vi "En Setting for Trig and LSL.vi"(9 "LSL En enum":enum16{"LSL Disabled", "LSL Enabled"}(ring), 10 "Soft Trig enum":T1(ring), 11 "Data Cluster in":T2) -> (3 "Data Cluster out":T2)   [LabVIEW 2019, in "CML UI.lvlib"]
uses:
  CML UI.lvlib
  Module Data--cluster.ctl
  Acquisition State.ctl
  Measurement UI Displays.ctl
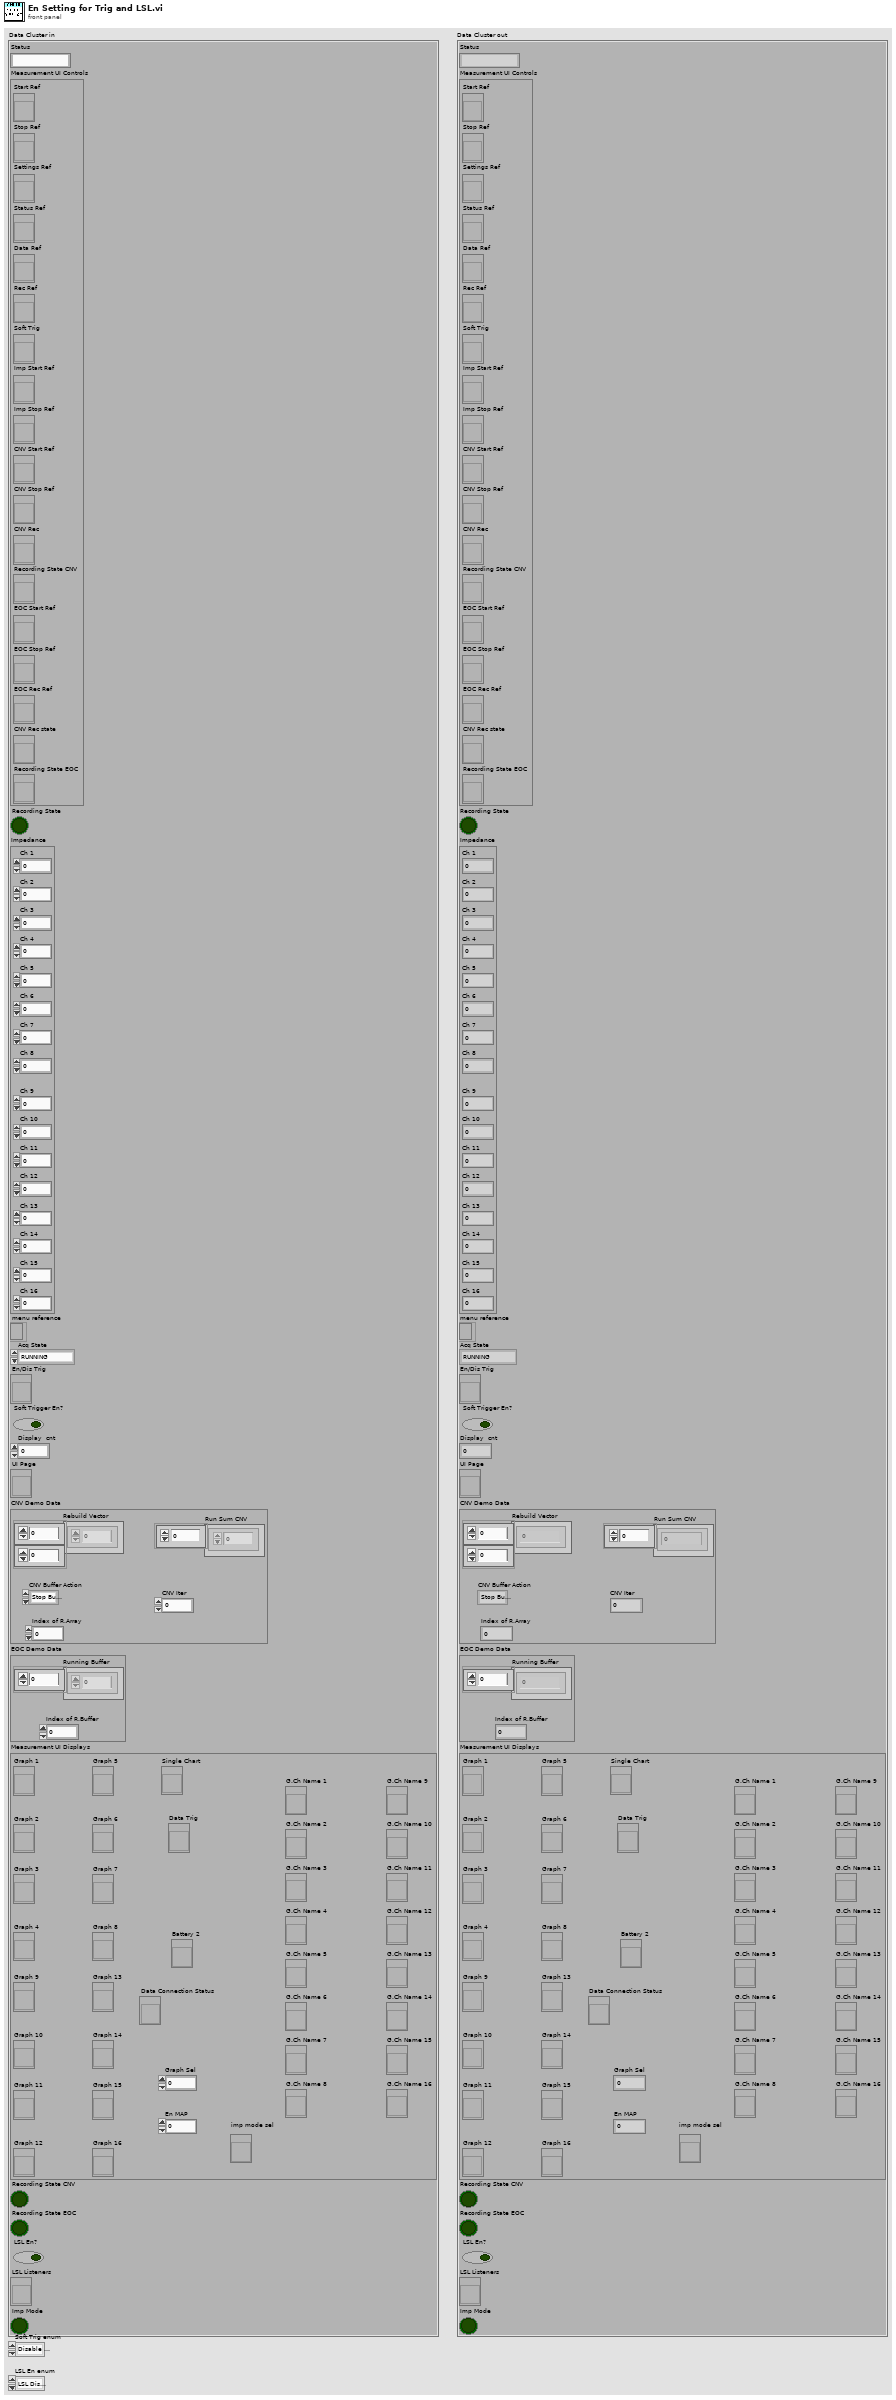
[diagram p1: front panel]
types:
  T1 = enum16{"Disable Soft Trigger", "Enable Soft Trigger"}
  T2 = typedef "CML UI.lvlib/Module Data--cluster.ctl" = cluster{"Status":string, "Measurement UI Controls":cluster{"Start Ref":refnum<vi>, "Stop Ref":refnum<vi>, "Settings Ref":refnum<vi>, "Status Ref":refnum<vi>, "Data Ref":refnum<vi>, "Rec Ref":refnum<vi>, "Soft Trig":refnum<vi>, "Imp Start Ref":refnum<vi>, "Imp Stop Ref":refnum<vi>, "CNV Start Ref":refnum<vi>, "CNV Stop Ref":refnum<vi>, "CNV Rec":refnum<vi>, "Recording State CNV":refnum<vi>, "EOC Start Ref":refnum<vi>, "EOC Stop Ref":refnum<vi>, "EOC Rec Ref":refnum<vi>, "CNV Rec state":refnum<vi>, "Recording State EOC":refnum<vi>}, "Recording State":bool, "Impedance":cluster{"Ch 1":dbl, "Ch 2":dbl, "Ch 3":dbl, "Ch 4":dbl, "Ch 5":dbl, "Ch 6":dbl, "Ch 7":dbl, "Ch 8":dbl, "Ch 9":dbl, "Ch 10":dbl, "Ch 11":dbl, "Ch 12":dbl, "Ch 13":dbl, "Ch 14":dbl, "Ch 15":dbl, "Ch 16":dbl}, "menu reference ":refnum<k9>, "Acq State":T3, "En/Dis Trig":refnum<vi>, "Soft Trigger En?":bool, "Display  cnt":u8, "UI Page":refnum<vi>, "CNV Demo Data":cluster{"Rebuild Vector":dbl[][], "CNV Buffer Action":enum16{"Stop Buffer Fill", "Start Buffer Fill", "Analyze Buffer"}, "Index of R.Array":u16, "Run Sum CNV":dbl[], "CNV Iter":u16}, "EOC Demo Data":cluster{"Running Buffer":dbl[], "Index of R.Buffer":u8}, "Measurement UI Displays":T4, "Recording State CNV":bool, "Recording State EOC":bool, "LSL En?":bool, "LSL Listeners":refnum<vi>, "Imp Mode":bool}
  T3 = typedef "CML UI.lvlib/Acquisition State.ctl" = enum16{"RUNNING", "IDLE"}
  T4 = typedef "CML UI.lvlib/Measurement UI Displays.ctl" = cluster{"Graph 1":refnum<vi>, "Graph 2":refnum<vi>, "Graph 3":refnum<vi>, "Graph 4":refnum<vi>, "Graph 5":refnum<vi>, "Graph 6":refnum<vi>, "Graph 7":refnum<vi>, "Graph 8":refnum<vi>, "Graph 9":refnum<vi>, "Graph 10":refnum<vi>, "Graph 11":refnum<vi>, "Graph 12":refnum<vi>, "Graph 13":refnum<vi>, "Graph 14":refnum<vi>, "Graph 15":refnum<vi>, "Graph 16":refnum<vi>, "Battery 2":refnum<vi>, "Data Trig":refnum<vi>, "Data Connection Status":refnum<vi>, "Graph Sel":u8, "En MAP":u16, "Single Chart":refnum<vi>, "G.Ch Name 1":refnum<vi>, "G.Ch Name 2":refnum<vi>, "G.Ch Name 3":refnum<vi>, "G.Ch Name 4":refnum<vi>, "G.Ch Name 5":refnum<vi>, "G.Ch Name 6":refnum<vi>, "G.Ch Name 7":refnum<vi>, "G.Ch Name 8":refnum<vi>, "G.Ch Name 9":refnum<vi>, "G.Ch Name 10":refnum<vi>, "G.Ch Name 11":refnum<vi>, "G.Ch Name 12":refnum<vi>, "G.Ch Name 13":refnum<vi>, "G.Ch Name 14":refnum<vi>, "G.Ch Name 15":refnum<vi>, "G.Ch Name 16":refnum<vi>, "imp mode sel":refnum<vi>}
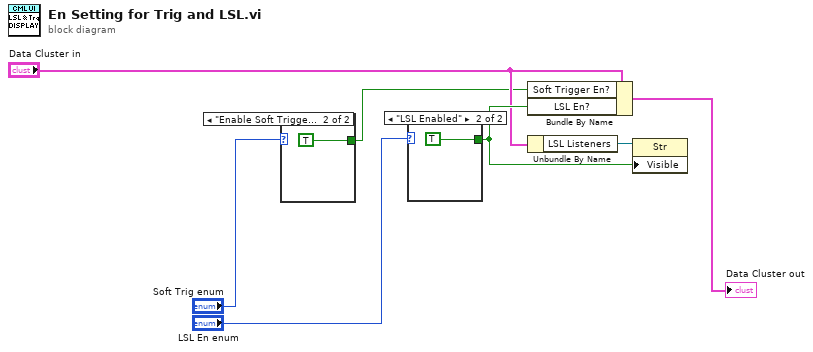
[diagram p0: block diagram]
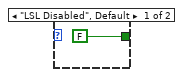
[diagram p2: hidden frame]
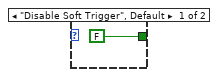
[diagram p3: hidden frame]
diagram:
  n1 = case shown="\"Enable Soft Trigger\"" "Soft Trig enum" {
    tunnel: [FALSE TRUE] -> w2
    frame "Disable Soft Trigger", Default {
    }
    frame "Enable Soft Trigger" {
    }
  }
  n2 = case shown="\"LSL Enabled\"" "LSL En enum" {
    tunnel: [FALSE TRUE] -> w6
    frame "LSL Disabled", Default {
    }
    frame "LSL Enabled" {
    }
  }
  n3 = Bundle By Name(cluster="Data Cluster in", "Soft Trigger En?"=w2, "LSL En?"=w6) -> (→"Data Cluster out":T2)
  n4 = Unbundle By Name("Data Cluster in") -> ("LSL Listeners"=w5:refnum<vi>)
  n5 = property class="Str"(reference=w5, "Visible"=w6) -> ()  [unwired: 1 in, 2 out]
